vi "Write DIO.vi"(11 "Generator Data in":T1) -> ()   [LabVIEW 2016]
uses:
  Typedefs/Generator Data Cluster.ctl
  <vilib>/rvi/eio/common/nirviEmuTemplateMethod_errors.vi
  <vilib>/eio/EIONode/EIONode.xnode
  Host/Typedefs/IO Buffer Operation.ctl
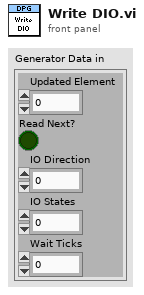
[diagram p1: front panel]
types:
  T1 = typedef "Generator Data Cluster.ctl" = cluster{"Updated Element":u64, "Read Next?":bool, "IO Direction":u32, "IO States":u32, "Wait Ticks":u32}
  T2 = typedef "IO Buffer Operation.ctl" = enum16{"Initialize", "Write IO Data_Rd", "Read IO Data_Rd", "Write IO Data_Wr", "Read IO Data_Wr", "Write  IO Data_Dir", "Read  IO Data_Dir", "Write Host to Target FIFO", "Read Host to Target FIFO", "Write Target to Host FIFO", "Read Target to Host FIFO", "Write Monitor Enable?", "Read Monitor Enable?", "Close"}
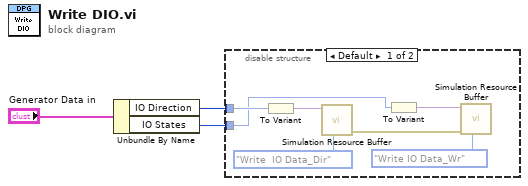
[diagram p0: block diagram]
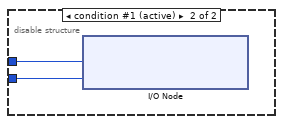
[diagram p2: hidden frame]
diagram:
  n1 = Unbundle By Name("Generator Data in") -> ("IO Direction"=w2:u32, "IO States"=w1:u32)
  n2 = disable-structure shown="Default" {
    disable-tunnel: w2 -> [w9 w12]
    disable-tunnel: w1 -> [w4 w11]
    frame condition #0 {
      n3 = To Variant(anything=w9) -> (Variant=w8:variant)
      n4 = call "Simulation Resource Buffer.vi"("IO Buffer Operation"=IO_Buffer_Operation."Write  IO Data_Dir", "Data in"=w8) -> ("error out"=w5:errorcluster)  [unwired: 7 in, 2 out]
      n5 = To Variant(anything=w4) -> (Variant=w6:variant)
      n6 = call "Simulation Resource Buffer.vi"("IO Buffer Operation"=IO_Buffer_Operation."Write IO Data_Wr", "error in (no error)"=w5, "Data in"=w6) -> ()  [unwired: 6 in, 3 out]
    }
    frame condition #1 (active) {
      n7 = xnode "I/O Node"("IO Module\\SE_Data_Dir"=w12, "IO Module\\SE_Data_Wr"=w11) -> ()  [unwired: 2 in, 2 out]
    }
  }
